vi "Init.vi"() -> (3 "Notifier Transport out":refnum<class "Notifier Transport.lvclass">)   [LabVIEW 2025, in "jettl.lvlib" / "Transport.lvlib" / "Notifier.lvlib" / "Notifier Transport.lvclass"]
uses:
  Notifier Transport.lvclass
  Notifier Transport.lvclass/Notifier Transport.ctl
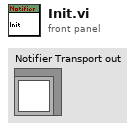
[diagram p1: front panel]
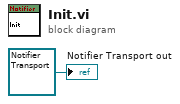
[diagram p0: block diagram]
diagram:
  "Notifier Transport out" <- refnum<class "Notifier Transport.lvclass"> refnum ("Notifier Transport out")
